vi "SACAR_NOMBRE.vi"(10 "Array 2":string[](array[string])) -> (3 "deleted portion":string)   [LabVIEW 2015]
panel:
  out "reversed array":string[](array[string])
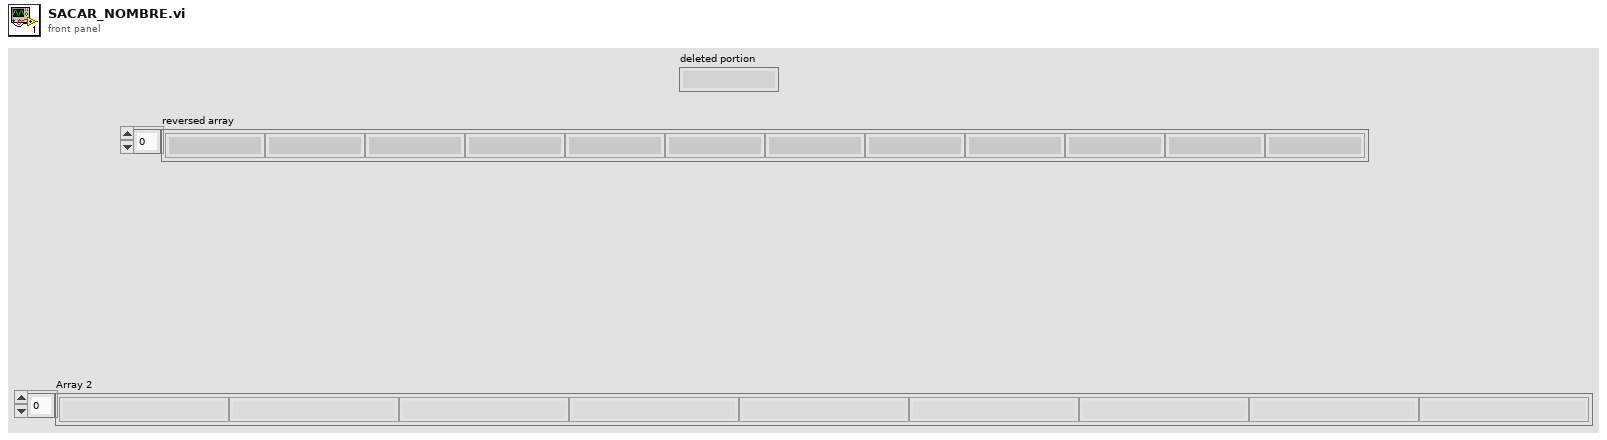
[diagram p1: front panel]
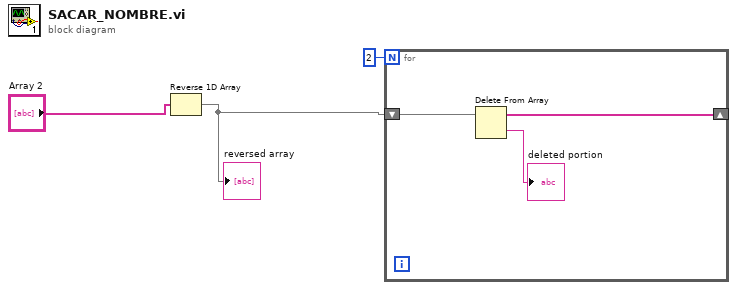
[diagram p0: block diagram]
diagram:
  n1 = Reverse 1D Array(array="Array 2") -> (reversed array=w1:string[])
  "reversed array" <- w1
  n2 = for {
    N: 2 -> [_]
    shift-right: [w5] -> _
    shift-left: w1 -> [w6]
    n3 = Delete From Array(array=w6) -> (deleted portion=→"deleted portion":string, array with subset deleted=w5:string[])  [unwired: 2 in]
  }
